vi "HDI Start Position Acquire.vi"() -> ()   [LabVIEW 2011]
uses:
  Shared Components/Orient3d Class/Type Definitions/Quaternion.ctl
  Shared Components/Gantry Class/Gantry Class.lvclass
  Shared Components/Vec3d Class/Vec3d Class.lvclass
  Shared Components/Orient3d Class/Orient3d Class.lvclass
panel:
  in  "Tab Control":enum32{"Control", "Results"}(tab)
  out "error out":errorcluster
  out "preview":T1(plugin-control)
  out "Current Position":cluster{"X":dbl, "Y":dbl, "Z":dbl}
  in  "Slot Number":i32
  in  "Capture":bool
  in  "Config Folder":path=path "C:/Users/Husker/Desktop/gantry/Config"
  out "Orientation":T2
  out "Center":cluster{"X":dbl, "Y":dbl, "Z":dbl}
  out "Residual":dbl
  out "Measured Positions":cluster{"X":dbl, "Y":dbl, "Z":dbl}[](array[cluster])
  out "Known Positions":cluster{"X":dbl, "Y":dbl, "Z":dbl}[](array[cluster])
  out "DoCapture":bool
  # "Set this to the appropriate slot number before running"
  # "Press this button after \ncentering the fiducial in the image"
  # "After aquiring positions, place these results in\npart_location.ini under the HDI heading"
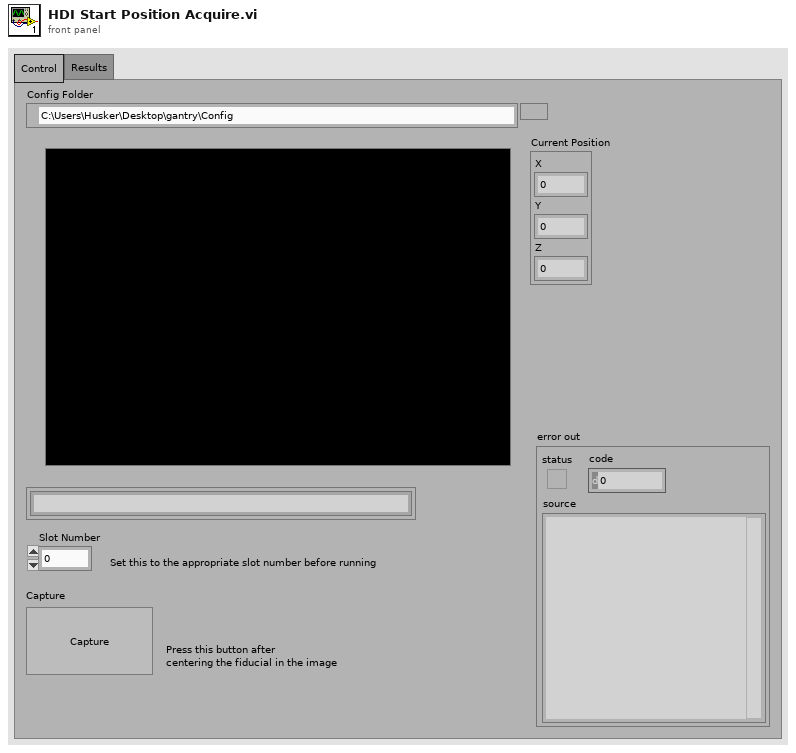
[diagram p1: front panel]
types:
  T1 = typedef "IMAQ Image.ctl" = refnum<image>
  T2 = typedef "Quaternion.ctl" = cluster{"x":dbl, "y":dbl, "z":dbl, "w":dbl}
  T3 = typedef "Image Type" = u32
  T4 = typedef "Position_Orientation.ctl" = cluster{"Center":refnum<class "Vec3d Class.lvclass">, "Orientation":refnum<class "Orient3d Class.lvclass">}
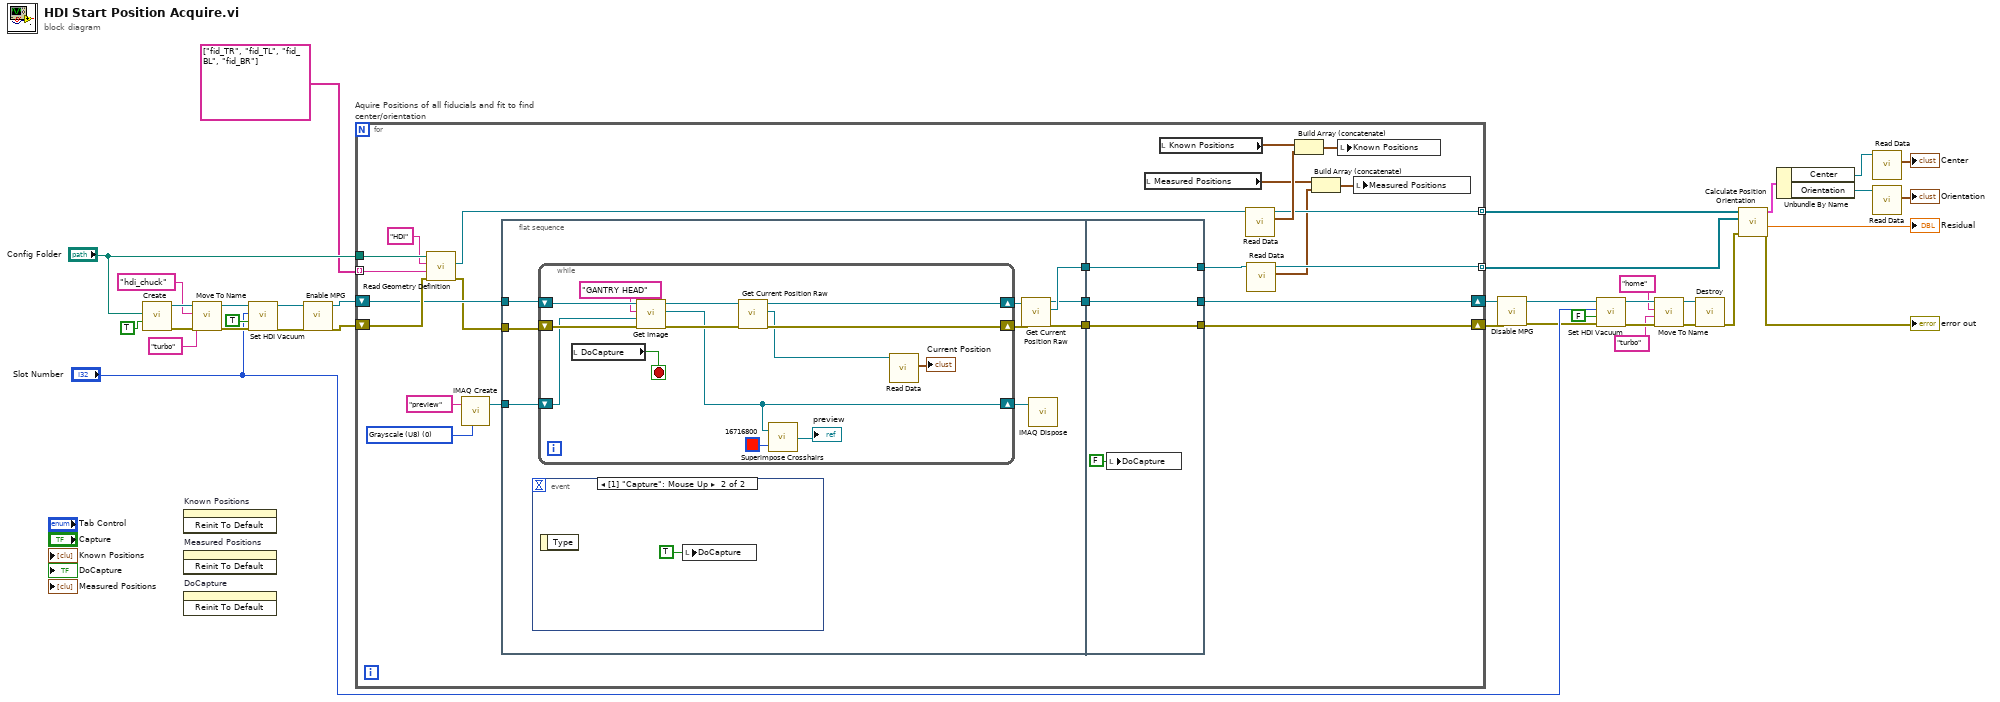
[diagram p0: block diagram]
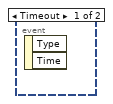
[diagram p2: hidden frame]
diagram:
  n1 = call "Create.vi"("HOME?"=TRUE, "Config Folder"="Config Folder") -> ("error out"=w17:errorcluster, "Gantry out"=w15:refnum<class "Gantry Class.lvclass">)  [unwired: 8 in]
  n2 = invoke on="Known Positions" class="Arr (strict)" method="Reinit To Default"() -> ()  [unwired: 3 in, 3 out]
  n3 = invoke on="Measured Positions" class="Arr (strict)" method="Reinit To Default"() -> ()  [unwired: 3 in, 3 out]
  n4 = invoke on="DoCapture" class="Bool (strict)" method="Reinit To Default"() -> ()  [unwired: 3 in, 3 out]
  n5 = call-dynamic "Move To Name.vi"("error in"=w17, "Speeds Label"="turbo", "Destination Name"="hdi_chuck", "Gantry in"=w15) -> ("error out"=w16:errorcluster, "Gantry out"=w14:refnum<class "Gantry Class.lvclass">)  [unwired: 6 in]
  n6 = call-dynamic "Set HDI Vacuum.vi"("error in"=w16, "On/Off"=TRUE, "Slot Number"="Slot Number", "Gantry in"=w14) -> ("error out"=w30:errorcluster, "Gantry out"=w32:refnum<class "Gantry Class.lvclass">)  [unwired: 6 in]
  n7 = call-dynamic "Enable MPG.vi"("error in (no error)"=w30, "Gantry Class in"=w32) -> ("error out"=w29:errorcluster, "Gantry Class out"=w31:refnum<class "Gantry Class.lvclass">)  [unwired: 8 in]
  n8 = for "Aquire Positions of all fiducials and fit to find center/orientation" {
    tunnel: "Config Folder" -> [w60]
    tunnel: string[] ["fid_TR", "fid_TL", "fid_BL", "fid_BR"] -> [w58] mode=indexing
    tunnel: [w45] -> w26 mode=indexing
    tunnel: [w43] -> w25 mode=indexing
    shift-right: [w54] -> w28
    shift-left: w31 -> [w56]
    shift-right: [w53] -> w27
    shift-left: w29 -> [w57]
    w38 = T3 0 items=["Grayscale (U8)", "Grayscale (I16)", "Grayscale (SGL)", "Complex (CSG)", "RGB (U32)", "HSL (U32)", "RGB (U64)", "Grayscale (U16)"] ("Image Type")
    n9 = call "Read Geometry Definition.vi"("error in"=w57, "Feature"=w58, "Part"="HDI", "Config Location"=w60) -> ("error out"=w55:errorcluster, "Feature Coordinates"=w49:refnum<class "Vec3d Class.lvclass">)  [unwired: 6 in]
    n10 = call "IMAQ Create"("Image Name"="preview", "Image Type"=w38) -> ("New Image"=w37:T1)  [unwired: 3 in, 1 out]
    n11 = flat-sequence {
      tunnel: w56 -> [w69]
      tunnel: w55 -> [w68]
      tunnel: [w65] -> w52
      tunnel: [w64] -> w51
      tunnel: [w63] -> w50
      tunnel: w37 -> [w62]
      tunnel: [w86] -> w53
      tunnel: [w87] -> w54
      tunnel: [w88] -> w44
      tunnel: w52 -> [w88]
      tunnel: w51 -> [w87]
      tunnel: w50 -> [w86]
      frame #0 {
        n12 = event shown="[1] \"Capture\": Mouse Up" {
          selector: _ -> [_ _]
          dyn-events: _ -> [_ _]
          timeout: _ -> [_ _]
          event Timeout {
            n13 = event-data() -> ()  [unwired: 1 in, 2 out]
          }
          event "Capture": Mouse Up {
            n14 = event-data() -> ()  [unwired: 1 in, 1 out]
            n15 = local write "DoCapture"(TRUE ("DoCapture")) -> ()
          }
        }
        n16 = while {
          shift-right: [w77] -> w67
          shift-left: w68 -> [w82]
          shift-right: [w78] -> w66
          shift-left: w69 -> [w83]
          shift-right: [w71] -> w61
          shift-left: w62 -> [w72]
          stop <- w84 stop-if-true
          n17 = local read "DoCapture"() -> (w84:bool)
          n18 = call-dynamic "Get Image.vi"("error in"=w82, "Image In"=w72, "Camera Name"="GANTRY HEAD", "Gantry in"=w83) -> ("error out"=w79:errorcluster, "Image Out"=w71:T1, "Gantry out"=w80:refnum<class "Gantry Class.lvclass">)  [unwired: 5 in]
          n19 = call-dynamic "Get Current Position Raw.vi"("error in (no error)"=w79, "Gantry Class in"=w80) -> ("error out"=w77:errorcluster, "Vec3d Class out"=w76:refnum<class "Vec3d Class.lvclass">, "Gantry Class out"=w78:refnum<class "Gantry Class.lvclass">)  [unwired: 7 in]
          n20 = call "Superimpose Crosshairs.vi"("Grid Line Color"=u32 16716800, "Refnum in"=w71) -> ("Refnum out"=→"preview":T1)
          n21 = call-dynamic "Read Data.vi"("Vec3d Class in"=w76) -> ("Data"=→"Current Position":cluster{"X":dbl, "Y":dbl, "Z":dbl})  [unwired: 8 in, 2 out]
        }
        n22 = call-dynamic "Get Current Position Raw.vi"("error in (no error)"=w67, "Gantry Class in"=w66) -> ("error out"=w63:errorcluster, "Vec3d Class out"=w65:refnum<class "Vec3d Class.lvclass">, "Gantry Class out"=w64:refnum<class "Gantry Class.lvclass">)  [unwired: 7 in]
        n23 = call "IMAQ Dispose"("Image"=w61) -> ()  [unwired: 5 in, 1 out]
      }
      frame #1 {
        n24 = local write "DoCapture"(FALSE ("DoCapture")) -> ()
      }
    }
    n25 = local read "Measured Positions"() -> (w42:cluster{"X":dbl, "Y":dbl, "Z":dbl}[])
    n26 = local read "Known Positions"() -> (w48:cluster{"X":dbl, "Y":dbl, "Z":dbl}[])
    n27 = call-dynamic "Read Data.vi"("Vec3d Class in"=w49) -> ("Data"=w47:cluster{"X":dbl, "Y":dbl, "Z":dbl}, "Vec3d Class out"=w45:refnum<class "Vec3d Class.lvclass">)  [unwired: 8 in, 1 out]
    n28 = call-dynamic "Read Data.vi"("Vec3d Class in"=w44) -> ("Data"=w40:cluster{"X":dbl, "Y":dbl, "Z":dbl}, "Vec3d Class out"=w43:refnum<class "Vec3d Class.lvclass">)  [unwired: 8 in, 1 out]
    n29 = Build Array (concatenate)(w48, w47) -> (w46:cluster{"X":dbl, "Y":dbl, "Z":dbl}[])
    n30 = Build Array (concatenate)(w42, w40) -> (w41:cluster{"X":dbl, "Y":dbl, "Z":dbl}[])
    n31 = local write "Known Positions"(w46) -> ()
    n32 = local write "Measured Positions"(w41) -> ()
  }
  n33 = call-dynamic "Disable MPG.vi"("error in (no error)"=w27, "Gantry Class in"=w28) -> ("error out"=w9:errorcluster, "Gantry Class out"=w11:refnum<class "Gantry Class.lvclass">)  [unwired: 8 in]
  n34 = call-dynamic "Set HDI Vacuum.vi"("error in"=w9, "On/Off"=FALSE, "Slot Number"="Slot Number", "Gantry in"=w11) -> ("error out"=w4:errorcluster, "Gantry out"=w6:refnum<class "Gantry Class.lvclass">)  [unwired: 6 in]
  n35 = call-dynamic "Move To Name.vi"("error in"=w4, "Speeds Label"="turbo", "Destination Name"="home", "Gantry in"=w6) -> ("error out"=w3:errorcluster, "Gantry out"=w5:refnum<class "Gantry Class.lvclass">)  [unwired: 6 in]
  n36 = call "Destroy.vi"("error in"=w3, "Gantry Class in"=w5) -> ("error out"=w8:errorcluster)  [unwired: 9 in]
  n37 = call "Calculate Position Orientation.vi"("error in"=w8, "Measured Global Positions"=w25, "Known Local Positions"=w26) -> ("error out"=→"error out":errorcluster, "Residual"=→"Residual":dbl, "PositionOrientation"=w22:T4)  [unwired: 6 in]
  n38 = Unbundle By Name(w22) -> ("Center"=w21:refnum<class "Vec3d Class.lvclass">, "Orientation"=w19:refnum<class "Orient3d Class.lvclass">)
  n39 = call-dynamic "Read Data.vi"("Vec3d Class in"=w21) -> ("Data"=→"Center":cluster{"X":dbl, "Y":dbl, "Z":dbl})  [unwired: 8 in, 2 out]
  n40 = call "Read Data.vi"("Orient3d in"=w19) -> ("Quaternion"=→"Orientation":T2)  [unwired: 8 in, 2 out]
